vi "Adjust_Seconds.vi"(9 "Coords":T1, 10 "Label":string, 11 "Seconds":i32 caption="Value in\nSeconds:") -> (0 "Cancelled":bool, 3 "Seconds_out":i32)   [LabVIEW 2016]
uses:
  <vilib>/Utility/miscctls.llb/LVPoint32TypeDef.ctl
  <vilib>/Utility/miscctls.llb/LVRectTypeDef.ctl
panel:
  out "Slide":u8(slide)
  in  "Hr":i32 caption="Hour"
  in  "Min":i32 min=-1 max=720 format="%02.0f"
  in  "Sec":i32 min=-1 max=43200 format="%02.0f"
  in  "Cancel Button":bool
  in  "OK Button":bool
  # "Adjust Timer Set Value for:"
  # ":"
  # ":"
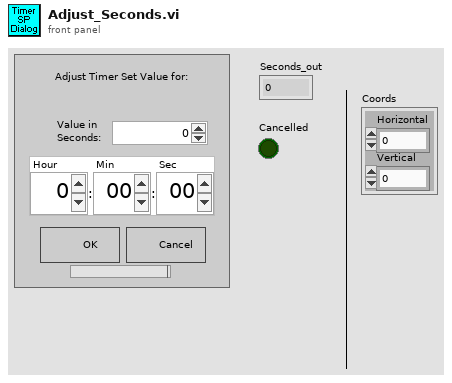
[diagram p1: front panel]
types:
  T1 = typedef "LVPoint32TypeDef.ctl" = cluster{"Horizontal":i32, "Vertical":i32}
  T2 = typedef "LVRectTypeDef.ctl" = cluster{"Left":i16, "Top":i16, "Right":i16, "Bottom":i16}
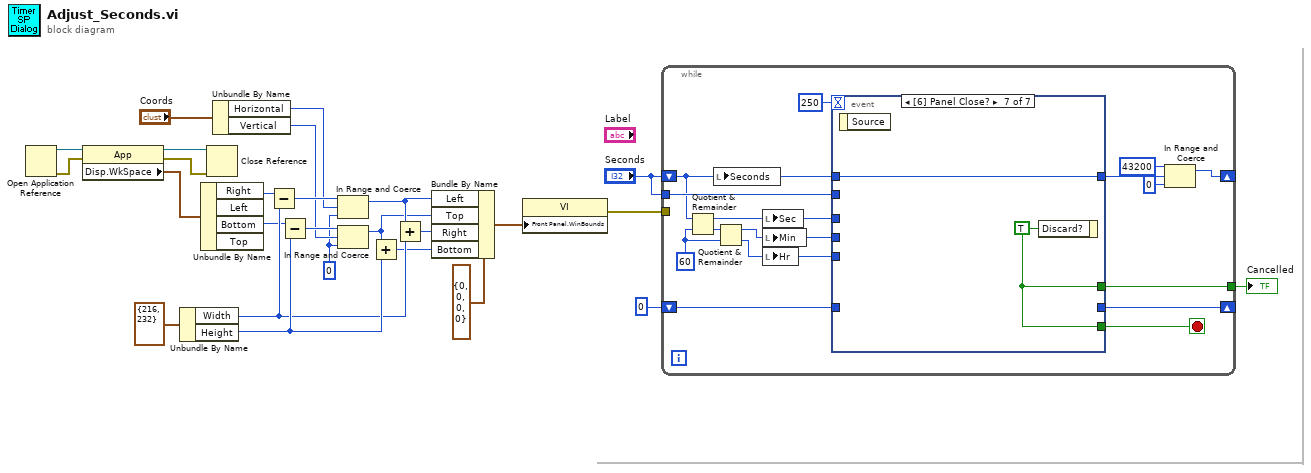
[diagram p0: block diagram]
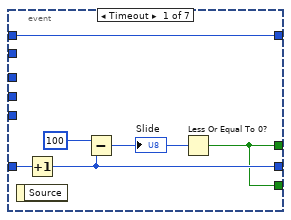
[diagram p2: hidden frame]
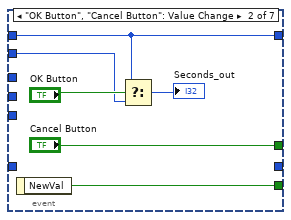
[diagram p3: hidden frame]
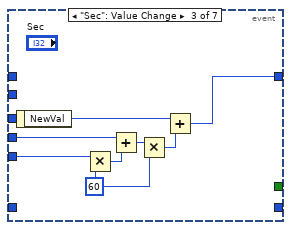
[diagram p4: hidden frame]
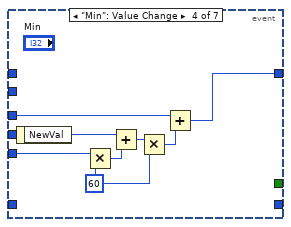
[diagram p5: hidden frame]
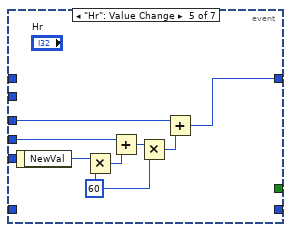
[diagram p6: hidden frame]
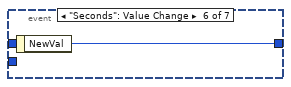
[diagram p7: hidden frame]
diagram:
  w9 = 0 ("lower limit")
  n1 = Open Application Reference() -> (0:w18:errorcluster, 3:w15:refnum<vi>)  [unwired: 1 in, 3 out]
  n2 = property class="App"(reference=w15, error in=w18) -> (reference out=w16:refnum<vi>, error out=w17:errorcluster, "Disp.WkSpace"=w19:T2)
  n3 = Unbundle By Name(cluster{"Width":i32, "Height":i32} {"Width"=216, "Height"=232} ("WindowSize")) -> ("Width"=w23:i32, "Height"=w24:i32)
  n4 = Unbundle By Name(w19) -> ("Right"=w20:i16, "Bottom"=w21:i16)  [unwired: 2 out]
  n5 = Close Reference(reference=w16, error in (no error)=w17) -> ()  [unwired: 1 out]
  n6 = Unbundle By Name("Coords") -> ("Horizontal"=w12:i32, "Vertical"=w10:i32)
  n7 = Subtract(x=w20, y=w23) -> (x-y=w13:i32)
  n8 = Subtract(x=w21, y=w24) -> (x-y=w11:i32)
  n9 = In Range and Coerce(upper limit=w13, x=w12, lower limit=w9) -> (coerced(x)=w8:i32)  [unwired: 1 out]
  n10 = In Range and Coerce(upper limit=w11, x=w10, lower limit=w9) -> (coerced(x)=w7:i32)  [unwired: 1 out]
  n11 = Add(x=w7, y=w24) -> (x+y=w5:i32)
  n12 = Add(x=w8, y=w23) -> (x+y=w6:i32)
  n13 = Bundle By Name(cluster=T2 {"Left"=0, "Top"=0, "Right"=0, "Bottom"=0} ("Front Panel Window:Window Bounds"), "Left"=w8, "Top"=w7, "Right"=w6, "Bottom"=w5) -> (w3:T2)
  n14 = property class="VI"("Front Panel.WinBounds"=w3) -> (error out=w2:errorcluster)  [unwired: 2 in, 1 out]
  n15 = while {
    shift-right: [w38] -> _
    shift-left: "Seconds" -> [w40]
    tunnel: "Seconds" -> [w41]
    tunnel: [w30] -> w25
    tunnel: w2 -> [_]
    shift-right: [w27] -> _
    shift-left: 0 -> [w28]
    stop <- w42 stop-if-true
    w34 = 60 ("y")
    n16 = Quotient & Remainder(x=w40, y=w34) -> (x-y*floor(x/y)=w32:i32, floor(x/y)=w35:i32)
    n17 = local write "Seconds"(w40) -> ()
    n18 = Quotient & Remainder(x=w35, y=w34) -> (x-y*floor(x/y)=w31:i32, floor(x/y)=w33:i32)
    n19 = local write "Sec"(w32) -> ()
    n20 = local write "Min"(w31) -> ()
    n21 = local write "Hr"(w33) -> ()
    n22 = event shown="[6] Panel Close?" {
      selector: _ -> [_ _ _ _ _ _ _]
      dyn-events: _ -> [_ _ _ _ _ _ _]
      timeout: 250 -> [_ _ _ _ _ _ _]
      tunnel: [w43 w54 _ _ _ _ w80] -> w42
      tunnel: [w48 w52 w61 w69 w77 w79 w81] -> w37
      tunnel: w40 -> [w48 w52 _ _ _ _ w81]
      tunnel: w41 -> [_ w51 _ _ _ _ _]
      tunnel: w33 -> [_ _ w56 w67 _ _ _]
      tunnel: w32 -> [_ _ _ w68 w73 _ _]
      tunnel: w31 -> [_ _ w59 _ w72 _ _]
      tunnel: [w43 "Cancel Button" _ _ _ _ w80] -> w30
      tunnel: w28 -> [w47 _ _ _ _ _ _]
      tunnel: [w45 _ _ _ _ _ _] -> w27
      event Timeout {
        n23 = event-data() -> ()  [unwired: 1 in, 1 out]
        n24 = Increment(x=w47) -> (x+1=w45:i32)
        n25 = Subtract(x=100, y=w45) -> (x-y=w44:i32)
        "Slide" <- w44
        n26 = Less Or Equal To 0?(x=w44) -> (x <= 0?=w43:bool)
      }
      event "OK Button", "Cancel Button": Value Change {
        n27 = event-data() -> ("NewVal"=w54:bool)  [unwired: 1 in]
        n28 = Select(t=w52, s="OK Button", f=w51) -> (s? t:f=→"Seconds_out":i32)
      }
      event "Sec": Value Change {
        w55 = 60 ("y")
        n29 = event-data() -> ("NewVal"=w60:i32)  [unwired: 1 in]
        n30 = Multiply(x=w56, y=w55) -> (x*y=w57:i32)
        n31 = Add(x=w59, y=w57) -> (x+y=w58:i32)
        n32 = Multiply(x=w58, y=w55) -> (x*y=w62:i32)
        n33 = Add(x=w60, y=w62) -> (x+y=w61:i32)
      }
      event "Min": Value Change {
        w66 = 60 ("y")
        n34 = event-data() -> ("NewVal"=w64:i32)  [unwired: 1 in]
        n35 = Multiply(x=w67, y=w66) -> (x*y=w65:i32)
        n36 = Add(x=w64, y=w65) -> (x+y=w63:i32)
        n37 = Multiply(x=w63, y=w66) -> (x*y=w70:i32)
        n38 = Add(x=w68, y=w70) -> (x+y=w69:i32)
      }
      event "Hr": Value Change {
        w74 = 60 ("y")
        n39 = event-data() -> ("NewVal"=w71:i32)  [unwired: 1 in]
        n40 = Multiply(x=w71, y=w74) -> (x*y=w75:i32)
        n41 = Add(x=w72, y=w75) -> (x+y=w76:i32)
        n42 = Multiply(x=w76, y=w74) -> (x*y=w78:i32)
        n43 = Add(x=w73, y=w78) -> (x+y=w77:i32)
      }
      event "Seconds": Value Change {
        n44 = event-data() -> ("NewVal"=w79:i32)  [unwired: 1 in]
      }
      event Panel Close? {
        w80 = TRUE ("Discard?")
        n45 = event-data() -> ()  [unwired: 1 in, 1 out]
        n46 = event-data("Discard?"=w80) -> ()  [unwired: 1 in, 1 out]
      }
    }
    n47 = In Range and Coerce(upper limit=43200, x=w37, lower limit=0) -> (coerced(x)=w38:i32)  [unwired: 1 out]
  }
  "Cancelled" <- w25
